vi "Reset.vi"(8 "error in (no error)":errorcluster, 11 "State Machine in":refnum<class "State Machine.lvclass">) -> (0 "error out":errorcluster, 3 "State Machine out":refnum<class "State Machine.lvclass">)   [LabVIEW 2018, in "State Machine.lvclass"]
doc: "Este VI reseta a máquina de estados."
uses:
  State Machine.lvclass
  State Machine.lvclass/State Machine.ctl
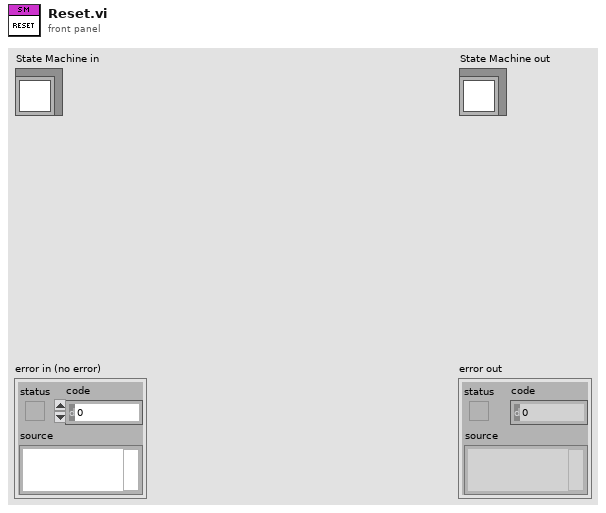
[diagram p1: front panel]
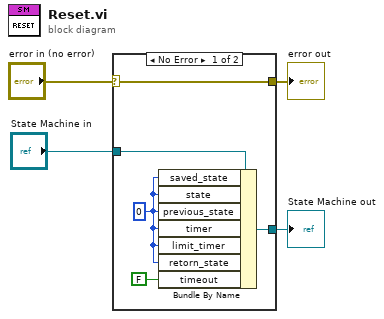
[diagram p0: block diagram]
diagram:
  n1 = case shown="No Error" "error in (no error)" {
    selector: "error in (no error)" -> [w9 w11]
    tunnel: [w9 w11] -> w3
    tunnel: [w5 w10] -> w1
    tunnel: "State Machine in" -> [w6 w10]
    frame No Error {
      w7 = u32 0
      n2 = Bundle By Name(cluster=w6, "saved_state"=w7, "state"=w7, "previous_state"=w7, "timer"=w7, "limit_timer"=w7, "retorn_state"=w7, "timeout"=FALSE) -> (w5:refnum<class "State Machine.lvclass">)
    }
    frame Error {
    }
  }
  "error out" <- w3
  "State Machine out" <- w1
